vi "ExSubAsyncColDispStrGblQ.vi"(2 "error in (no error)":errorcluster, 3 "Store Data":bool, 4 "Display Title":string, 5 "Handle Cluster":T1) -> (0 "error out":errorcluster, 1 "Handle Cluster Out":T1)   [LabVIEW 2010]
panel:
  # "ExSubAsyncColDispStr:\nThis Sub-VI does the data collection, \ndisplay, and storage for Async\ncamera operations."
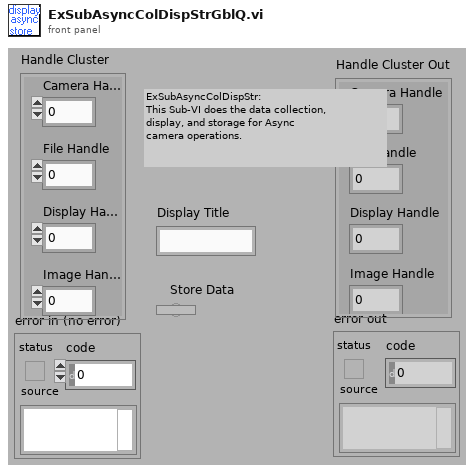
[diagram p1: front panel]
types:
  T1 = cluster{"Camera Handle":u32, "File Handle":u32, "Display Handle":u32, "Image Handle":u32}
  T2 = cluster{"Camera Handle":u32, "File Handle":u32, "Display Handle":u32, "Data Handle":u32}
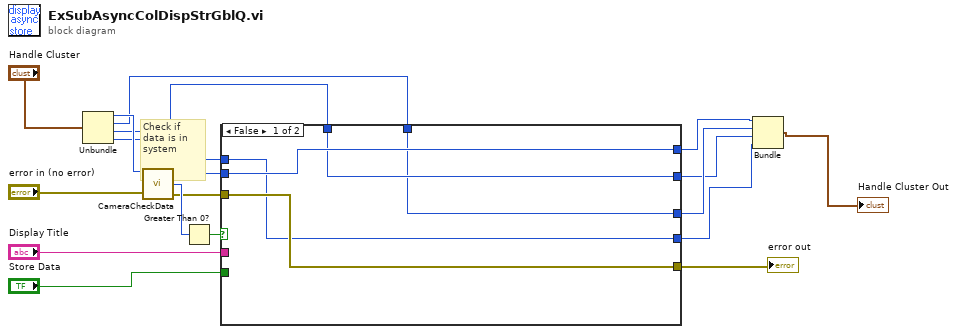
[diagram p0: block diagram]
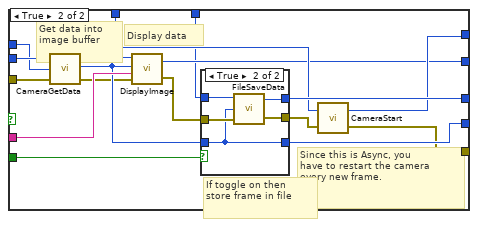
[diagram p2: hidden frame]
diagram:
  # "Check if \ndata is in\nsystem"
  n1 = Unbundle("Handle Cluster") -> ("Camera Handle"=w5:u32, "File Handle"=w3:u32, "Display Handle"=w2:u32, "Image Handle"=w4:u32)
  n2 = call <userlib>:"CameraCheckData.vi"("Camera Handle"=w5, "error in"="error in (no error)") -> ("Camera Handle"=w17:u32, "Number Of Frames Available"=w16:i32, "error out"=w15:errorcluster)
  n3 = Greater Than 0?(x=w16) -> (x > 0?=w18:bool)
  n4 = case shown="False" w18 {
    tunnel: w17 -> [w23 w40]
    tunnel: w15 -> [w22 w39]
    tunnel: w4 -> [w20 w37]
    tunnel: w2 -> [w21 w36]
    tunnel: [w23 w27] -> w10
    tunnel: [w19 w38] -> w8
    tunnel: "Display Title" -> [_ w35]
    tunnel: w3 -> [w19 w24]
    tunnel: [w21 w25] -> w7
    tunnel: [w22 w28] -> w12
    tunnel: [w20 w33] -> w6
    tunnel: "Store Data" -> [_ w32]
    frame False {
    }
    frame True {
      # "If toggle on then\nstore frame in file"
      # "Since this is Async, you\nhave to restart the camera\nevery new frame."
      # "Display data"
      # "Get data into\nimage buffer"
      n5 = call <userlib>:"CameraGetData.vi"("error in"=w39, "Data Handle"=w37, "Camera Handle"=w40) -> ("error out"=w31:errorcluster, "Data Handle"=w34:u32, "Camera Handle"=w26:u32)
      n6 = call <userlib>:"DisplayImage.vi"("error in"=w31, "Title"=w35, "Image Handle"=w34, "Display Handle"=w36) -> ("error out"=w30:errorcluster, "Display Handle"=w25:u32)
      n7 = case shown="True" w32 {
        tunnel: [w43 w48] -> w38
        tunnel: w30 -> [w42 w47]
        tunnel: w24 -> [w43 w44]
        tunnel: [w42 w46] -> w29
        tunnel: w34 -> [w41 w45]
        tunnel: [w41 w45] -> w33
        frame False {
        }
        frame True {
          n8 = call <userlib>:"FileSaveData.vi"("error in"=w47, "Image Handle"=w45, "File Handle"=w44) -> ("error out"=w46:errorcluster, "File Handle"=w48:u32)
        }
      }
      n9 = call <userlib>:"CameraStart.vi"("error in"=w29, "Camera Handle"=w26) -> ("error out"=w28:errorcluster, "Camera Handle"=w27:u32)
    }
  }
  "error out" <- w12
  n10 = Bundle("Camera Handle"=w10, "File Handle"=w8, "Display Handle"=w7, "Data Handle"=w6) -> (→"Handle Cluster Out":T2)  [unwired: 1 in]
